vi "Round up or down ToFixedDPs.vi"(6 "Round":enum16{"Up", "Down", "Nearest"}(ring), 9 "Power of ten":i32, 11 "Number to round":dbl=1234.56789 format="%_9f") -> (1 "Decimal place":dbl=1.0 format="%#_9f", 3 "Rounded number":dbl=1235.0 format="%_9f")   [LabVIEW 2021]
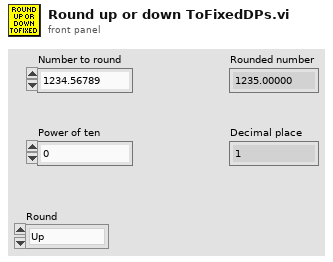
[diagram p1: front panel]
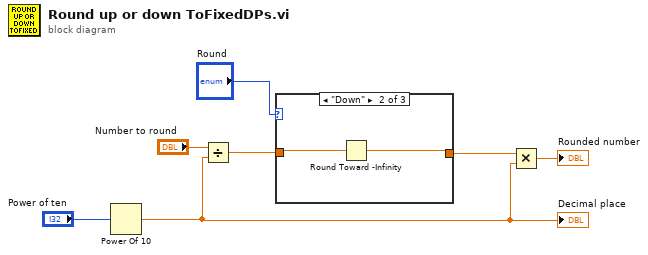
[diagram p0: block diagram]
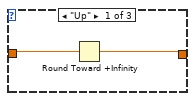
[diagram p2: hidden frame]
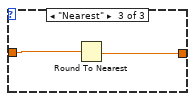
[diagram p3: hidden frame]
diagram:
  n1 = Power Of 10(x="Power of ten") -> (10^x=w7:dbl)
  "Decimal place" <- w7
  n2 = Divide(x="Number to round", y=w7) -> (x/y=w4:dbl)
  n3 = case shown="\"Down\"" "Round" {
    tunnel: [w8 w10 w13] -> w5
    tunnel: w4 -> [w9 w11 w12]
    frame "Up" {
      n4 = Round Toward +Infinity(x=w9) -> (ceil(x): smallest int >= x=w8:dbl)
    }
    frame "Down" {
      n5 = Round Toward -Infinity(1:w11) -> (0:w10:dbl)
    }
    frame "Nearest" {
      n6 = Round To Nearest(number=w12) -> (nearest integer value=w13:dbl)
    }
  }
  n7 = Multiply(x=w5, y=w7) -> (x*y=→"Rounded number":dbl)
